vi "control.by-index.vi"(8 "error in (no error)":errorcluster, 10 "control index":i32, 11 "VI in":refnum<vi>) -> (0 "error out":errorcluster, 2 "Ctl Refnum":refnum<vi>, 3 "VI out":refnum<vi>)   [LabVIEW 2020]
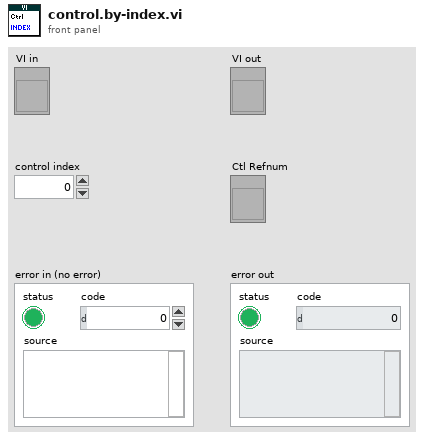
[diagram p1: front panel]
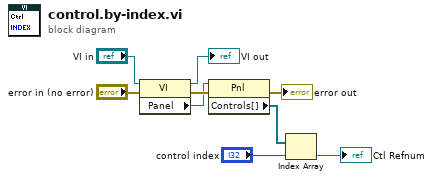
[diagram p0: block diagram]
diagram:
  n1 = property class="VI"(reference="VI in", error in="error in (no error)") -> (reference out=→"VI out":refnum<vi>, error out=w2:errorcluster, "Panel"=w1:refnum<vi>)
  n2 = property class="Pnl"(reference=w1, error in=w2) -> (error out=→"error out":errorcluster, "Controls[]"=w4:refnum<vi>[])  [unwired: 1 out]
  n3 = Index Array(array=w4, index="control index") -> (element=→"Ctl Refnum":refnum<vi>)
